vi "SMU Measure.vi"(8 "error in (no error)":errorcluster, 11 "SMU in":refnum<class "NI SMU.lvclass">) -> (0 "error out":errorcluster, 3 "SMU out":refnum<class "NI SMU.lvclass">)   [LabVIEW 2020, in "NI SMU.lvlib" / "NI SMU.lvclass"]
uses:
  NI SMU.lvclass
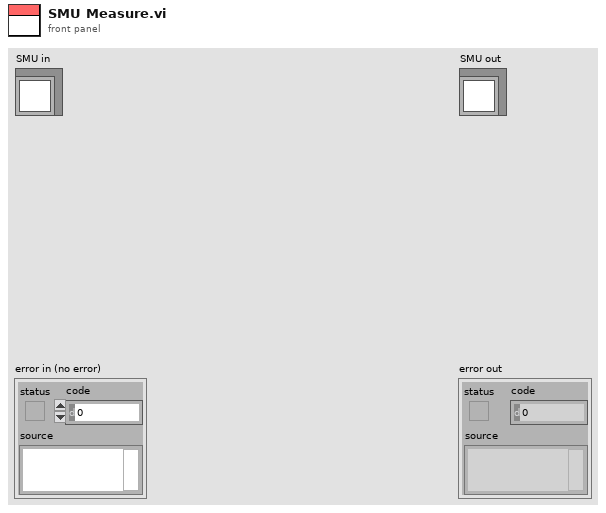
[diagram p1: front panel]
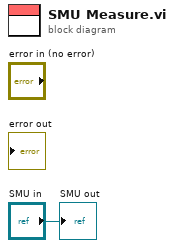
[diagram p0: block diagram]
diagram:
  "SMU out" <- "SMU in"
